vi "rspvtd_Get Settings.vi"(8 "error in":errorcluster, 11 "Data in":variant) -> (0 "error out":errorcluster, 3 "Data out":T1)   [LabVIEW 2023, in "Settings Window.lvclass"]
doc: "This VI converts variant data contained in the associated <b>Public API Response</b> message to its correct data type.\n---"
uses:
  Settings Window.lvclass
  rsp_Get Settings.ctl
  Settings.ctl
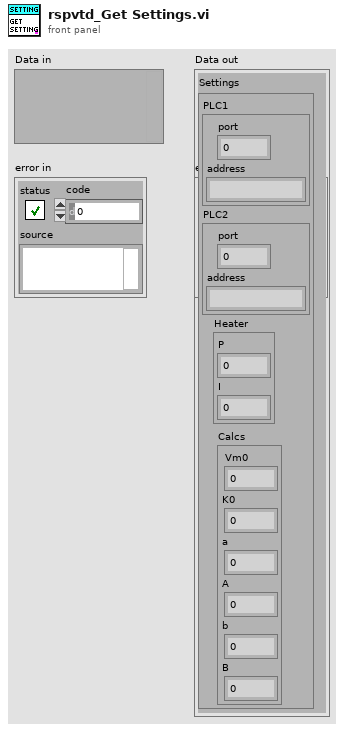
[diagram p1: front panel]
types:
  T1 = typedef "Settings Window.lvclass/rsp_Get Settings.ctl" = cluster{"Settings":T2}
  T2 = typedef "Settings Window.lvclass/Settings.ctl" = cluster{"PLC1":cluster{"port":u16, "address":string}, "PLC2":cluster{"port":u16, "address":string}, "Heater":cluster{"P":dbl, "I":dbl}, "Calcs":cluster{"Vm0":dbl, "K0":dbl, "a":dbl, "A":dbl, "b":dbl, "B":dbl}}
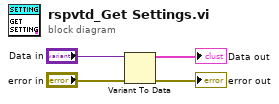
[diagram p0: block diagram]
diagram:
  n1 = Variant To Data(error in="error in", Variant="Data in") -> (data=→"Data out":T1, error out=→"error out":errorcluster)  [unwired: 1 in]
